vi "获取MAC地址.vi"(1 "英文系统":bool) -> (0 "MAC Address":string)   [LabVIEW 2018]
doc: "This VI uses the system exec VI to issue the command line utilities \"ping\" and \"arp\" to obtain the MAC Address of the network interface from a different computer on your network. Its functionality is limited to Windows systems.\n\nThe arp utility only works for IP addresses on the same local subnet as the computer executing the VI. Furthermore, it does not work for the IP address of the computer running the VI. This utility attempts to use the ipconfig utility for Windows NT/2000/XP to get the MAC Address of the local computer, but if the local computer's IP Address is given, it will fail when run under Windows 9x or Windows ME."
panel:
  out "standard output":string caption="标准输出"
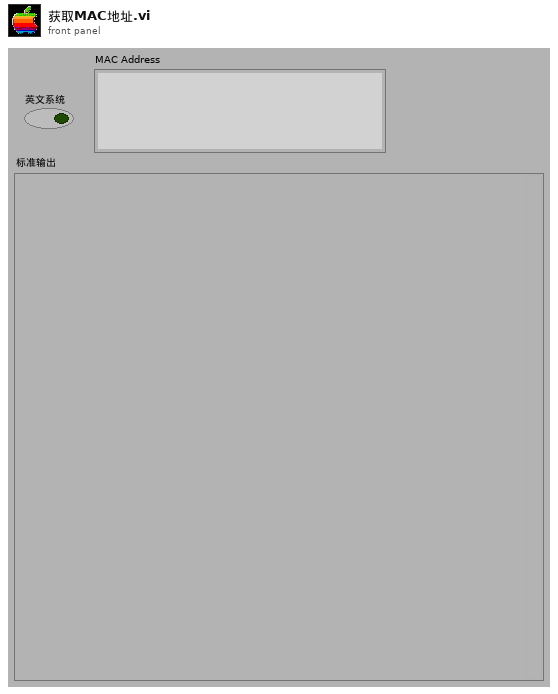
[diagram p1: front panel]
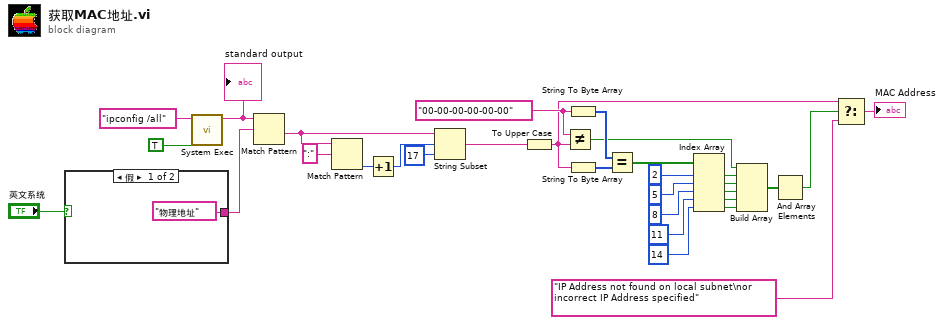
[diagram p0: block diagram]
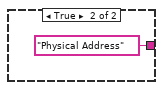
[diagram p2: hidden frame]
diagram:
  w15 = "00-00-00-00-00-00" ("regular expression")
  n1 = case shown="假" "英文系统" {
    tunnel: ["物理地址" ("regular expression") "Physical Address" ("regular expression")] -> w7
    frame False {
    }
    frame True {
    }
  }
  n2 = call <vilib>:"System Exec.vi"("run minimized? (F)"=TRUE, "command line"="ipconfig /all") -> ("standard output"=w8:string)  [unwired: 4 in, 5 out]
  "standard output" <- w8
  n3 = Match Pattern(string=w8, regular expression=w7) -> (after substring=w5:string)  [unwired: 4 out]
  n4 = Match Pattern(string=w5, regular expression=":") -> (offset past match=w4:i32)  [unwired: 4 out]
  n5 = Increment(x=w4) -> (x+1=w2:i32)
  n6 = String Subset(string=w5, offset (0)=w2, length (rest)=17 ("length (rest)")) -> (substring=w13:string)
  n7 = To Upper Case(1:w13) -> (0:w12:string)
  n8 = Not Equal?(x=w15, y=w12) -> (x != y?=w14:bool)
  n9 = String To Byte Array(string=w15) -> (unsigned byte array=w17:u8[])
  n10 = String To Byte Array(string=w12) -> (unsigned byte array=w16:u8[])
  n11 = Equal?(x=w17, y=w16) -> (x = y?=w18:bool[])
  n12 = Index Array(array=w18, index #1=2 ("index"), index #2=5 ("index"), index #3=8 ("index"), index #4=11 ("index"), index #5=14 ("index")) -> (element #1=w28:bool, element #2=w27:bool, element #3=w26:bool, element #4=w25:bool, element #5=w24:bool)
  n13 = Build Array(w14, w28, w27, w26, w25, w24) -> (w29:bool[])
  n14 = And Array Elements(Boolean array=w29) -> (logical AND=w30:bool)
  n15 = Select(t=w12, s=w30, f="IP Address not found on local subnet\nor incorrect IP Address specified") -> (s? t:f=→"MAC Address":string)
